vi "Impedance_Cryo_Configuration.vi"() -> ()   [LabVIEW 2018]
uses:
  <vilib>/Utility/file.llb/Write Delimited Spreadsheet (DBL).vi
  <instrlib>/Agilent 4194/Agilent 4194.lvlib
panel:
  in  "stop 2":bool
  in  "stop":bool
  in  "Start Impedance Collection":bool
  in  "Gain-Phase (0:Tch/Rch [dB] - Theta)":u32(ring) items=["Tch/Rch [dB] - Theta", "Tch/Rch - theta", "Tch/Rch [dB] - tau", "Tch-Rch [V]", "Tch-Rch [dBm]", "Tch-Rch [dBV]"]
  in  "Sweep Type (F:Linear)":bool
  in  "Stop/Span (10,00E-3)":dbl=15000000.0 format="%^.1e"
  in  "Start/Center (10,00E-3)":dbl=100.0 min=-40.0 max=40000000.0 format="%^.3e"
  in  "Display Mode (0:X - A&B)":u32(ring) items=["X - A&B", "A - B", "Table"]
  in  "Number Of Points (100)":i32=400 min=2 max=401
  in  "Averaging Number (8:256)":u32(ring) items=["1", "2", "4", "8", "16", "32", "64", "128", "256"]
  in  "Integration Time (0:Short)":u32(ring) items=["Short", "Medium", "Long"]
  in  "Impedance (0:| Z | - Theta )":u32(ring) items=["| Z | -Ttheta ", "R - X", "Ls-Rs", "Ls-Q", "Cs-Rs", "Cs-Q", "Cs-D", "|Y|-Theta", "G-B", "Lp-G", "Lp-Q", "Cp-G", "Cp-Q", "Cp-D", "|Z|-Ls", "|Z|-Cs", "|Z|-Lp", "|Z|-Cp", "Lp-Rp", "Cp-Rp"]
  in  "Measurement Type (0:Impedance)":u32(ring) items=["Impedance ", "Gain - Phase", "Impedance With Probe"]
  in  "File Base Name":string
  in  "error in (no error)":errorcluster
  in  "VISA resource name 2":refnum<visa-resource-name>="GPIB0::17::INSTR"
  out "A":T1(graph)
  out "B":T1(graph)
  out "error out":errorcluster
  in  "Force Quit":bool
  out "Status":string
  in  "Log Button In 4":bool
  in  "Log Button In 3":bool
  in  "Log Button In 2":bool
  in  "Log Button In 1":bool
  out "Input 4 Temperature Chart":dbl(graph)
  out "Input 3 Temperature Chart":dbl(graph)
  out "Input 1 Temperature Chart":dbl(graph)
  out "Input 2 Temperature Chart":dbl(graph)
  out "In 4 Value":dbl
  out "In 3 Value":dbl
  out "In 2 Value":dbl
  out "In 1 Value":dbl
  out "In 4 Channel Name":string
  out "In 3 Channel Name":string
  out "In 2 Channel Name":string
  out "In 1 Channel Name":string
  in  "VISA resource name":refnum<visa-resource-name>
  out "?":string
  out "?":string
  in  "Output 2":bool
  in  "Output 1":bool
  out "In 4 Channel Button Overlay":string
  out "In 3 Channel Button Overlay":string
  in  "Input 4 Button":bool
  in  "Input 3 Button":bool
  out "In 2 Channel Button Overlay":string
  out "In 1 Channel Button Overlay":string
  in  "Input 2 Button\nInput 2":bool
  in  "Input 1 Button":bool
  # "INPUT"
  # "OUTPUT"
  # "TEMPERATURE"
  # "K"
  # "K"
  # "K"
  # "K"
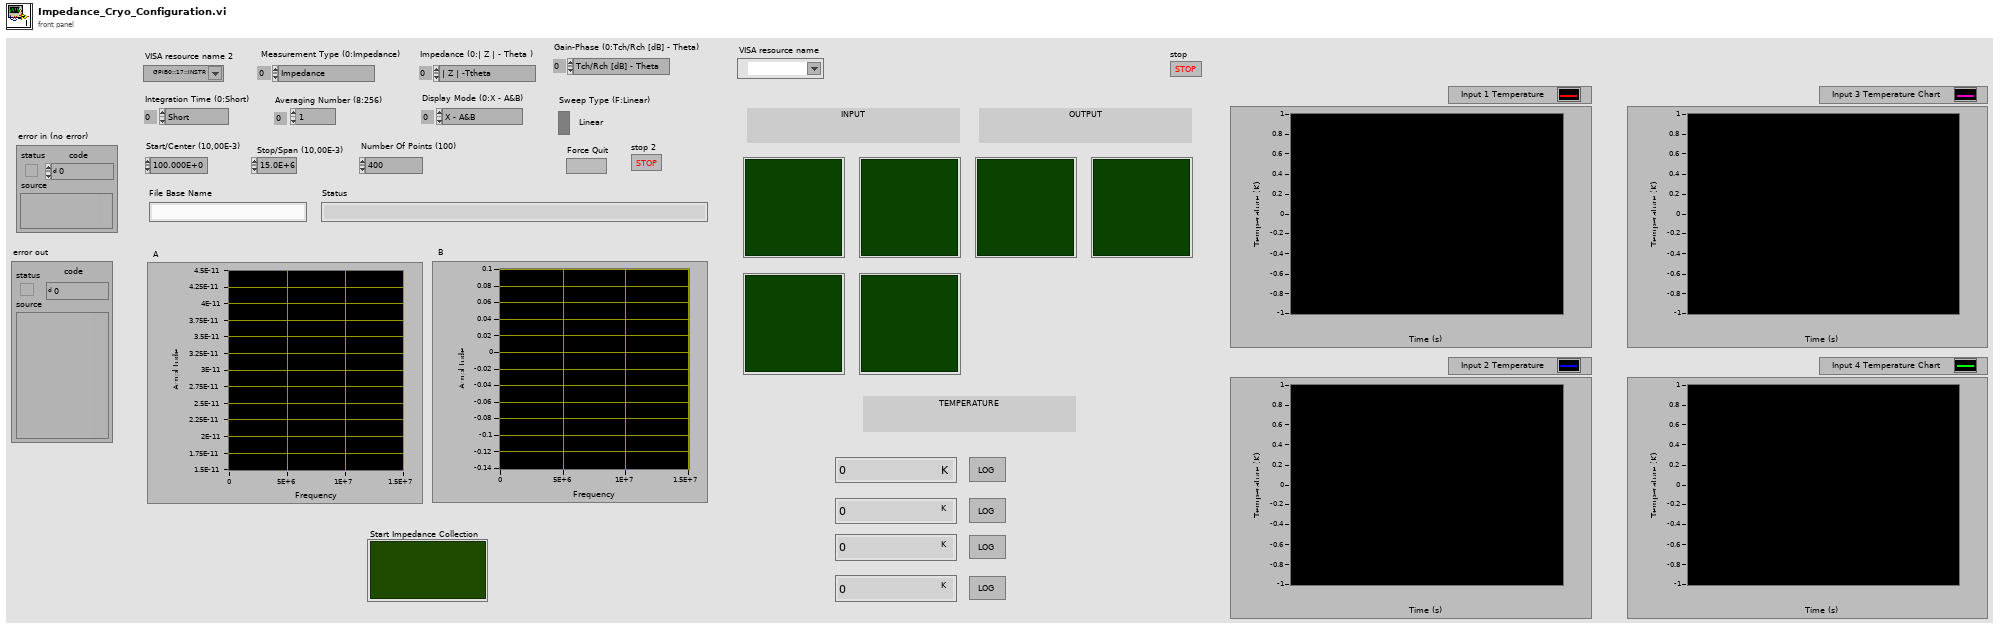
[diagram p1: front panel]
types:
  T1 = cluster{"Register Data":dbl[], "Offset/Calib Register Data":dbl[]}
  T2 = cluster{"[0]":dbl, "[1]":dbl, "[2]":dbl, "[3]":dbl, "[4]":dbl, "[5]":dbl, "[6]":dbl, "[7]":dbl, "[8]":dbl}
  T3 = cluster{"[0]":string, "[1]":string, "[2]":string, "[3]":string, "[4]":string, "[5]":string, "[6]":string, "[7]":string, "[8]":string}
  T4 = enum16{"open", "replace", "create", "open or create", "replace or create", "replace or create with confirmation"}
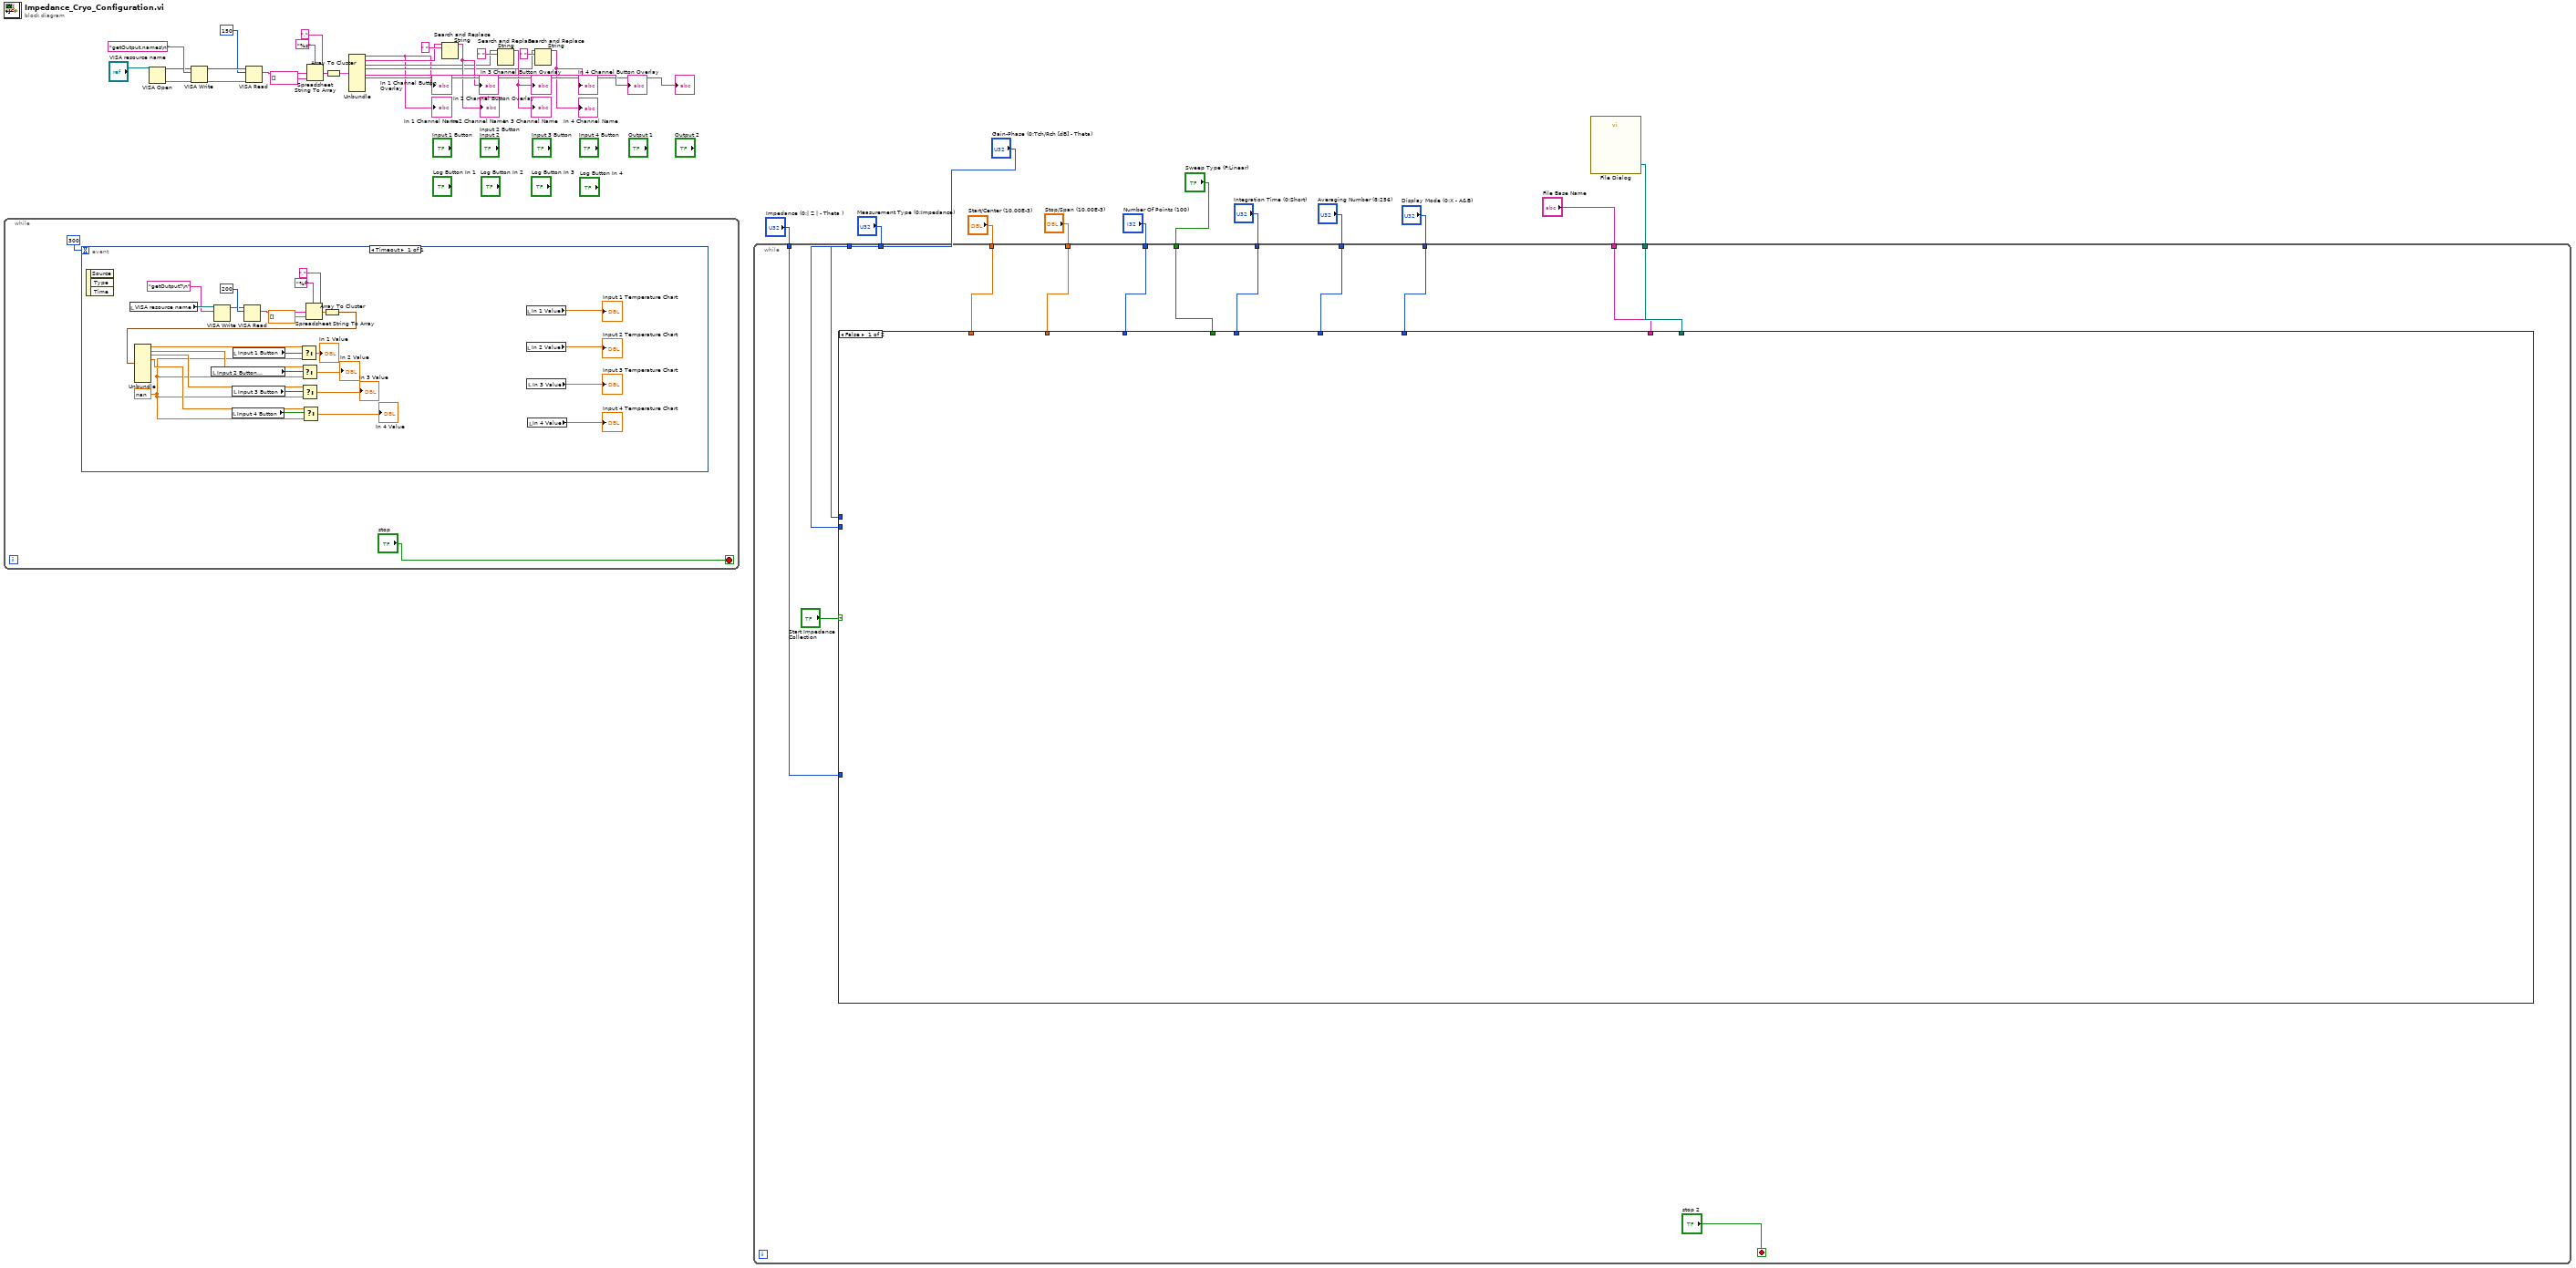
[diagram p0: block diagram]
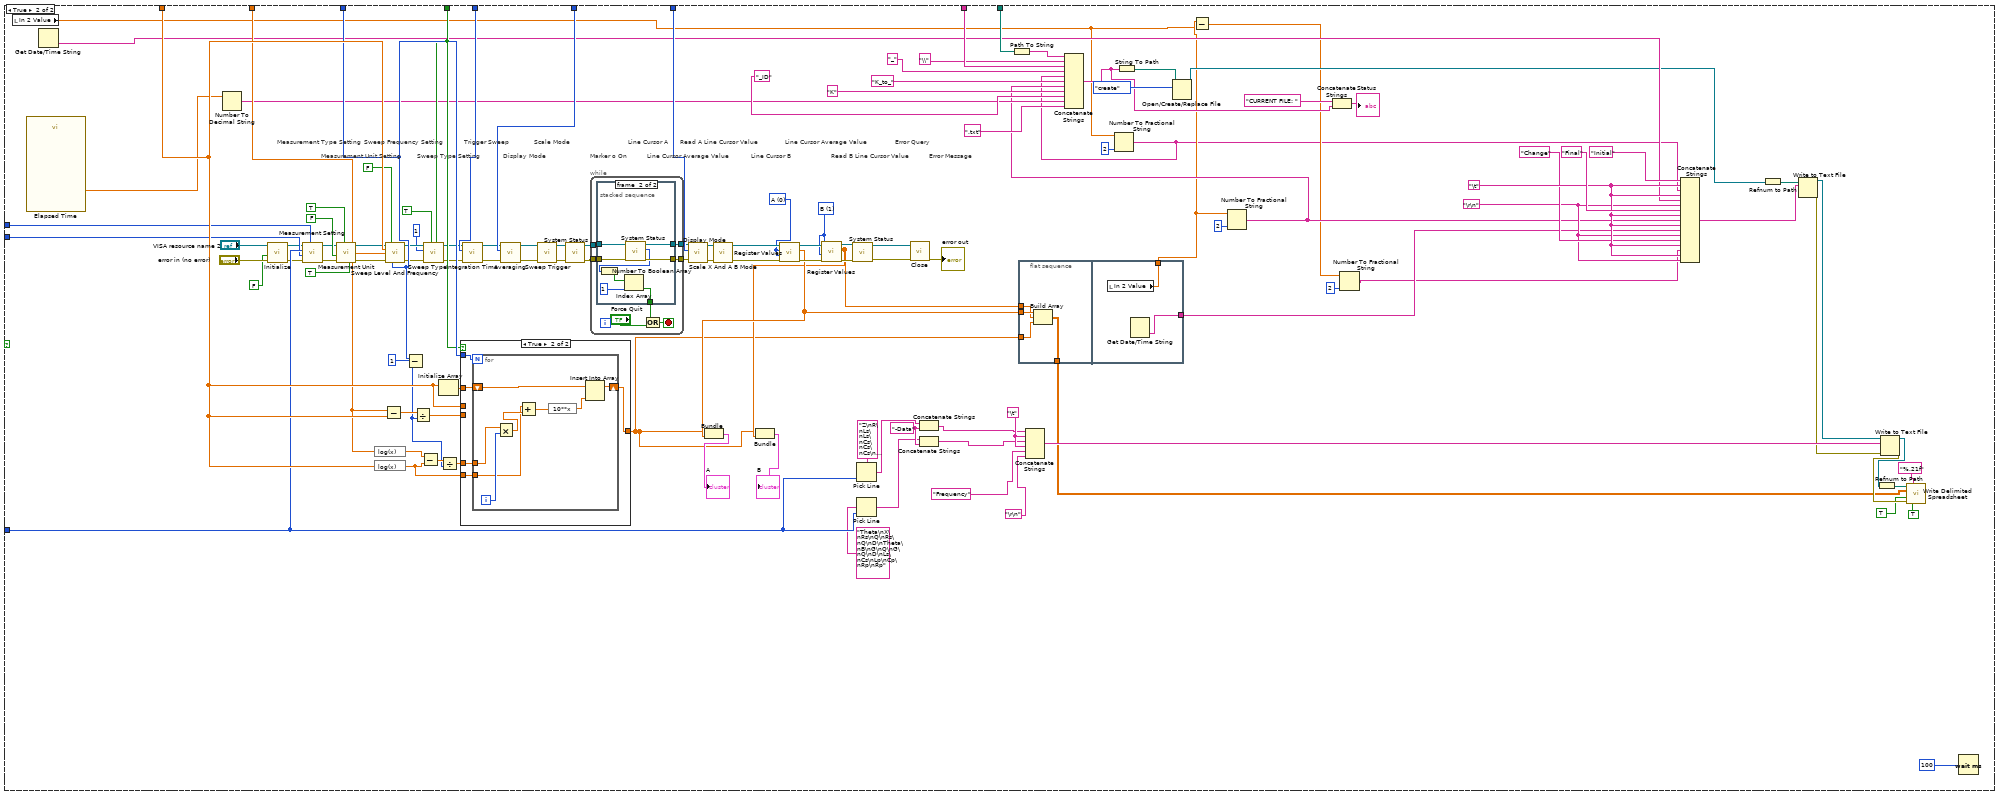
[diagram p2: hidden frame]
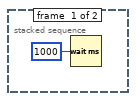
[diagram p3: hidden frame]
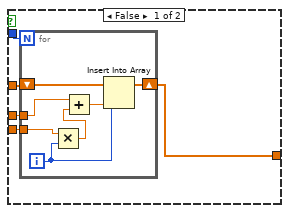
[diagram p4: hidden frame]
diagram:
  n1 = while {
    stop <- "stop" stop-if-true
    n2 = event shown="[0] Timeout" {
      selector: _ -> [_]
      dyn-events: _ -> [_]
      timeout: 300 -> [_]
      event Timeout {
        w49 = nan
        n3 = event-data() -> ()  [unwired: 1 in, 3 out]
        n4 = local read "VISA resource name"() -> (w66:refnum<visa-resource-name>)
        n5 = local read "Input 2 Button\nInput 2"() -> (w53:bool)
        n6 = VISA Write(VISA resource name=w66, write buffer="getOutput?\n") -> (VISA resource name out=w58:refnum<visa-resource-name>)  [unwired: 1 in, 2 out]
        n7 = local read "Input 4 Button"() -> (w48:bool)
        n8 = local read "Input 3 Button"() -> (w51:bool)
        n9 = local read "Input 1 Button"() -> (w55:bool)
        n10 = VISA Read(VISA resource name=w58, byte count=u32 200) -> (read buffer=w59:string)  [unwired: 1 in, 3 out]
        n11 = Spreadsheet String To Array(delimiter (Tab)=",", format string="%f", spreadsheet string=w59, array type (2D Dbl)=dbl[] []) -> (array=w61:dbl[])
        n12 = Array To Cluster(array=w61) -> (cluster=w57:T2)
        n13 = Unbundle(w57) -> ("[0]"=w56:dbl, "[1]"=w54:dbl, "[2]"=w52:dbl, "[3]"=w50:dbl)  [unwired: 5 out]
        n14 = Select(t=w56, s=w55, f=w49) -> (s? t:f=→"In 1 Value":dbl)
        n15 = Select(t=w54, s=w53, f=w49) -> (s? t:f=→"In 2 Value":dbl)
        n16 = Select(t=w52, s=w51, f=w49) -> (s? t:f=→"In 3 Value":dbl)
        n17 = Select(t=w50, s=w48, f=w49) -> (s? t:f=→"In 4 Value":dbl)
        n18 = local read "In 1 Value"() -> (→"Input 1 Temperature Chart":dbl)
        n19 = local read "In 2 Value"() -> (→"Input 2 Temperature Chart":dbl)
        n20 = local read "In 3 Value"() -> (→"Input 3 Temperature Chart":dbl)
        n21 = local read "In 4 Value"() -> (→"Input 4 Temperature Chart":dbl)
      }
    }
  }
  n22 = VISA Open(VISA resource name="VISA resource name") -> (VISA resource name=w13:refnum<visa-resource-name>, error out=w17:errorcluster)  [unwired: 4 in]
  n23 = VISA Write(VISA resource name=w13, write buffer="getOutput.names\n", error in (no error)=w17) -> (VISA resource name out=w20:refnum<visa-resource-name>, error out=w21:errorcluster)  [unwired: 1 out]
  n24 = VISA Read(VISA resource name=w20, byte count=u32 150, error in (no error)=w21) -> (read buffer=w15:string)  [unwired: 3 out]
  n25 = Spreadsheet String To Array(delimiter (Tab)=",", format string="%s", spreadsheet string=w15, array type (2D Dbl)=string[] []) -> (array=w31:string[])
  n26 = Array To Cluster(array=w31) -> (cluster=w34:T3)
  n27 = Unbundle(w34) -> ("[0]"=→"In 1 Channel Button Overlay" →"In 1 Channel Name":string, "[1]"=w29:string, "[2]"=w26:string, "[3]"=w23:string, "[4]"=→"?":string, "[5]"=→"?":string)  [unwired: 3 out]
  n28 = Search and Replace String(input string=w29, search string=" ") -> (result string=→"In 2 Channel Button Overlay" →"In 2 Channel Name":string)  [unwired: 6 in, 3 out]
  n29 = Search and Replace String(input string=w26, search string=" ") -> (result string=→"In 3 Channel Button Overlay" →"In 3 Channel Name":string)  [unwired: 6 in, 3 out]
  n30 = Search and Replace String(input string=w23, search string=" ") -> (result string=→"In 4 Channel Button Overlay" →"In 4 Channel Name":string)  [unwired: 6 in, 3 out]
  n31 = call "File Dialog"() -> ("selected path"=w5:path)  [unwired: 12 in, 3 out]
  n32 = while {
    tunnel: "Start/Center (10,00E-3)" -> [w80]
    tunnel: "Stop/Span (10,00E-3)" -> [w79]
    tunnel: "Number Of Points (100)" -> [w78]
    tunnel: "Sweep Type (F:Linear)" -> [w77]
    tunnel: "Integration Time (0:Short)" -> [w76]
    tunnel: "Averaging Number (8:256)" -> [w75]
    tunnel: "Display Mode (0:X - A&B)" -> [w74]
    tunnel: w5 -> [w73]
    tunnel: "File Base Name" -> [w72]
    tunnel: "Measurement Type (0:Impedance)" -> [w71]
    tunnel: "Impedance (0:| Z | - Theta )" -> [w70]
    tunnel: "Gain-Phase (0:Tch/Rch [dB] - Theta)" -> [w69]
    stop <- "stop 2" stop-if-true
    n33 = case shown="False" "Start Impedance Collection" {
      tunnel: w80 -> [_ w202]
      tunnel: w79 -> [_ w201]
      tunnel: w78 -> [_ w200]
      tunnel: w77 -> [_ w199]
      tunnel: w76 -> [_ w198]
      tunnel: w75 -> [_ w197]
      tunnel: w74 -> [_ w196]
      tunnel: w73 -> [_ w195]
      tunnel: w72 -> [_ w194]
      tunnel: w71 -> [_ w193]
      tunnel: w70 -> [_ w192]
      tunnel: w69 -> [_ w191]
      frame False {
      }
      frame True {
        w108 = "\r\n"
        w110 = "\t"
        w142 = "-Data" ("string")
        w145 = u32 0 items=["A", "B", "C", "D", "E", "F", "G", "H", "I", "J", "RA", "RB", "RC", "RD", "RE", "RF", "RG", "RH", "RI", "RJ", "RK", "RL"] ("Registers (0:A)")
        w149 = u32 1 items=["A", "B", "C", "D", "E", "F", "G", "H", "I", "J", "RA", "RB", "RC", "RD", "RE", "RF", "RG", "RH", "RI", "RJ", "RK", "RL"] ("Registers (0:A) 2")
        w148 = "\t"
        # "Error Message"
        # "Error Query"
        # "Line Cursor B"
        # "Line Cursor Average Value"
        # "Read B Line Cursor Value"
        # "Read A Line Cursor Value"
        # "Line Cursor Average Value"
        # "Line Cursor A"
        # "Marker o On"
        # "Scale Mode"
        # "Display Mode"
        # "Trigger Sweep"
        # "Sweep Type Setting"
        # "Sweep Frequency Setting"
        # "Measurement Unit Setting"
        # "Measurement Type Setting"
        n34 = local read "In 2 Value"() -> (w83:dbl)
        n35 = call "Elapsed Time"() -> ("Elapsed Time (s)"=w102:dbl)  [unwired: 12 in, 7 out]
        n36 = Get Date/Time String() -> (time string=w107:string)  [unwired: 3 in, 1 out]
        n37 = Number To Decimal String(number=w102) -> (decimal integer string=w98:string)  [unwired: 1 in]
        n38 = call <instrlib>:"Initialize.vi"("error in (no error)"="error in (no error)", "Reset Device (T:Reset Device)"=FALSE, "VISA resource name"="VISA resource name 2") -> ("error out"=w177:errorcluster, "VISA resource name out"=w176:refnum<visa-resource-name>)  [unwired: 7 in]
        n39 = call <instrlib>:"Measurement Setting.vi"("Measurement Type (0:Impedance)"=w193, "error in (no error)"=w177, "Gain-Phase (0:Tch/Rch [dB] - Theta)"=w191, "Impedance (0:| Z | - Theta )"=w192, "VISA resource name"=w176) -> ("error out"=w186:errorcluster, "VISA resource name out"=w187:refnum<visa-resource-name>)  [unwired: 5 in]
        n40 = call <instrlib>:"Measurement Unit.vi"("Test Input Impedance(T:50 ohm)"=TRUE ("Ref Attenuation (F:0 dB)"), "Power Splitter (F:Dual)"=TRUE ("Ref Attenuation (F:0 dB)"), "error in (no error)"=w186, "Ref Input Impedance (T:50 ohm)"=FALSE ("Ref Attenuation (F:0 dB)"), "VISA resource name"=w187) -> ("error out"=w184:errorcluster, "VISA resource name out"=w185:refnum<visa-resource-name>)  [unwired: 5 in]
        n41 = expression code="log(x)"(w201) -> (w155:dbl)
        n42 = expression code="log(x)"(w202) -> (w152:dbl)
        n43 = Subtract(x=w201, y=w202) -> (x-y=w165:dbl)
        n44 = call <instrlib>:"Sweep Level And Frequency.vi"("VISA resource name"=w185, "Step/Number Of Points (F:Points)"=FALSE ("Step/Number Of Points (F:Points))"), "Start/Center (10,00E-3)"=w202, "Stop/Span (10,00E-3)"=w201, "error in (no error)"=w184, "Number Of Points (100)"=w200) -> ("VISA resource name out"=w182:refnum<visa-resource-name>, "error out"=w181:errorcluster)  [unwired: 8 in]
        n45 = Subtract(x=w200, y=1) -> (x-y=w150:i32)
        n46 = Divide(x=w165, y=w150) -> (x/y=w164:dbl)
        n47 = Subtract(x=w155, y=w152) -> (x-y=w154:dbl)
        n48 = call <instrlib>:"Sweep Type.vi"("Sweep Type (F:Linear)"=w199, "Sweep Direction (F:Down)"=TRUE, "error in (no error)"=w181, "Sweep Mode (0:Repeat)"=u32 1, "VISA resource name"=w182) -> ("error out"=w172:errorcluster, "VISA resource name out"=w173:refnum<visa-resource-name>)  [unwired: 5 in]
        n49 = Initialize Array(w202) -> (w166:dbl[])  [unwired: 1 in]
        n50 = Divide(x=w154, y=w150) -> (x/y=w153:dbl)
        n51 = case shown="True" w199 {
          tunnel: w166 -> [w229 w240]
          tunnel: w200 -> [w228 w241]
          tunnel: w164 -> [w227 _]
          tunnel: w202 -> [w226 _]
          tunnel: [w225 w239] -> w92
          tunnel: w153 -> [_ w238]
          tunnel: w152 -> [_ w237]
          frame False {
            n52 = for {
              N: w228 -> [_]
              shift-right: [w235] -> w225
              shift-left: w229 -> [w236]
              tunnel: w226 -> [w232]
              tunnel: w227 -> [w230]
              i -> [w234]
              n53 = Multiply(x=w230, y=w234) -> (x*y=w231:dbl)
              n54 = Add(x=w232, y=w231) -> (x+y=w233:dbl)
              n55 = Insert Into Array(array=w236, index=w234, new element=w233) -> (w235:dbl[])
            }
          }
          frame True {
            n56 = for {
              N: w241 -> [_]
              shift-right: [w249] -> w239
              shift-left: w240 -> [w248]
              tunnel: w238 -> [w246]
              tunnel: w237 -> [w242]
              i -> [w245]
              n57 = Multiply(x=w246, y=w245) -> (x*y=w247:dbl)
              n58 = Add(x=w242, y=w247) -> (x+y=w244:dbl)
              n59 = expression code="10**x"(w244) -> (w243:dbl)
              n60 = Insert Into Array(array=w248, new element=w243) -> (w249:dbl[])  [unwired: 1 in]
            }
          }
        }
        n61 = call <instrlib>:"Integration Time.vi"("error in (no error)"=w172, "Integration Time (0:Short)"=w198, "VISA resource name"=w173) -> ("error out"=w170:errorcluster, "VISA resource name out"=w171:refnum<visa-resource-name>)  [unwired: 7 in]
        n62 = call <instrlib>:"Averaging.vi"("error in (no error)"=w170, "Averaging Number (8:256)"=w197, "VISA resource name"=w171) -> ("error out"=w168:errorcluster, "VISA resource name out"=w169:refnum<visa-resource-name>)  [unwired: 7 in]
        n63 = call <instrlib>:"Sweep Trigger.vi"("error in (no error)"=w168, "VISA resource name"=w169) -> ("error out"=w134:errorcluster, "VISA resource name out"=w135:refnum<visa-resource-name>)  [unwired: 8 in]
        n64 = call <instrlib>:"System Status.vi"("error in (no error)"=w134, "VISA resource name"=w135) -> ("error out"=w133:errorcluster, "VISA resource name out"=w132:refnum<visa-resource-name>)  [unwired: 6 in, 2 out]
        n65 = while {
          tunnel: w132 -> [w215]
          tunnel: w133 -> [w214]
          tunnel: [w213] -> w137
          tunnel: [w212] -> w136
          stop <- w211 stop-if-true
          n66 = stacked-sequence {
            tunnel: w215 -> [_ w224]
            tunnel: w214 -> [_ w223]
            tunnel: [_ w222] -> w213
            tunnel: [_ w221] -> w212
            tunnel: [_ w220] -> w209
            frame #0 {
              n67 = Wait (ms)(milliseconds to wait=u32 1000) -> ()  [unwired: 1 out]
            }
            frame #1 {
              n68 = call <instrlib>:"System Status.vi"("error in (no error)"=w223, "VISA resource name"=w224) -> ("error out"=w221:errorcluster, "ESR? (0)"=w219:i32, "VISA resource name out"=w222:refnum<visa-resource-name>)  [unwired: 6 in, 1 out]
              n69 = Number To Boolean Array(number=w219) -> (Boolean array=w218:bool[])
              n70 = Index Array(array=w218, index=1) -> (element=w220:bool)
            }
          }
          n71 = Or(x=w209, y="Force Quit") -> (x .or. y?=w211:bool)
        }
        n72 = call <instrlib>:"Display Mode.vi"("error in (no error)"=w136, "Display Mode (0:X - A&B)"=w196, "VISA resource name"=w137) -> ("error out"=w178:errorcluster, "VISA resource name out"=w179:refnum<visa-resource-name>)  [unwired: 7 in]
        n73 = call <instrlib>:"Scale X And A B Mode.vi"("VISA resource name"=w179, "error in (no error)"=w178) -> ("VISA resource name out"=w160:refnum<visa-resource-name>, "error out"=w159:errorcluster)  [unwired: 12 in]
        n74 = call <instrlib>:"Register Values.vi"("error in (no error)"=w159, "Calib/Offset Register (0:OFSTA)"=w145, "Registers (0:A)"=w145, "VISA resource name"=w160) -> ("error out"=w157:errorcluster, "Register Data"=w94:dbl[], "VISA resource name out"=w158:refnum<visa-resource-name>)  [unwired: 2 in, 3 out]
        n75 = Bundle(w92, "Register Data"=w94) -> (→"A":cluster{dbl[], "Register Data":dbl[]})  [unwired: 1 in]
        n76 = call <instrlib>:"Register Values.vi"("error in (no error)"=w157, "Calib/Offset Register (0:OFSTA)"=w149, "Registers (0:A)"=w149, "VISA resource name"=w158) -> ("error out"=w130:errorcluster, "Register Data"=w93:dbl[], "VISA resource name out"=w131:refnum<visa-resource-name>)  [unwired: 2 in, 3 out]
        n77 = Bundle(w92, "Register Data"=w93) -> (→"B":cluster{dbl[], "Register Data":dbl[]})  [unwired: 1 in]
        n78 = call <instrlib>:"System Status.vi"("error in (no error)"=w130, "VISA resource name"=w131) -> ("error out"=w128:errorcluster, "VISA resource name out"=w129:refnum<visa-resource-name>)  [unwired: 6 in, 2 out]
        n79 = Pick Line(multi-line string="Z\nR\nLs\nLs\nCs\nCs\nCs\nY\nG\nLp\nLp\nCp\nCp\nCp\nZ\nZ\nZ\nZ\nLp\nCp", line index=w192) -> (output string=w141:string)  [unwired: 1 in]
        n80 = Pick Line(multi-line string="Theta\nX\nRs\nQ\nRs\nQ\nD\nTheta\nB\nG\nQ\nG\nQ\nD\nLs\nCs\nLp\nCp\nRp\nRp", line index=w192) -> (output string=w140:string)  [unwired: 1 in]
        n81 = call <instrlib>:"Close.vi"("error in (no error)"=w128, "VISA resource name"=w129) -> ("error out"=→"error out":errorcluster)  [unwired: 9 in]
        n82 = Concatenate Strings(w141, w142) -> (w139:string)
        n83 = Concatenate Strings(w140, w142) -> (w138:string)
        n84 = Path To String(path=w195) -> (string=w127:string)
        n85 = flat-sequence {
          tunnel: w94 -> [w206]
          tunnel: w93 -> [w205]
          tunnel: w92 -> [w204]
          tunnel: [w203] -> w91
          tunnel: [w208] -> w88
          tunnel: [w207] -> w90
          frame #0 {
            n86 = Build Array(w206, w205, w204) -> (w203:dbl[][])
          }
          frame #1 {
            n87 = local read "In 2 Value"() -> (w208:dbl)
            n88 = Get Date/Time String() -> (time string=w207:string)  [unwired: 3 in, 1 out]
          }
        }
        n89 = Concatenate Strings(w139, w148, w138, w148, "Frequency" ("string"), "\r\n") -> (w117:string)
        n90 = Number To Fractional String(number=w83, precision (6)=i16 2) -> (F-format string=w82:string)  [unwired: 2 in]
        n91 = Subtract(x=w88, y=w83) -> (x-y=w85:dbl)
        n92 = Number To Fractional String(number=w88, precision (6)=i16 2) -> (F-format string=w89:string)  [unwired: 2 in]
        n93 = Concatenate Strings(w127, "\\", w194, "_", w82, "K_to_" ("string"), w89, "K" ("string"), "_ID", w98, ".txt" ("string")) -> (w95:string)
        n94 = String To Path(string=w95) -> (path=w125:path)
        n95 = Open/Create/Replace File(file path (use dialog)=w125, operation (0:open)=T4."create") -> (refnum out=w106:refnum<file>)  [unwired: 4 in, 2 out]
        n96 = Concatenate Strings("CURRENT FILE: " ("string"), w95) -> (→"Status":string)
        n97 = Number To Fractional String(number=w85, precision (6)=i16 2) -> (F-format string=w86:string)  [unwired: 2 in]
        n98 = Concatenate Strings("Initial" ("string"), w110, w82, w110, w107, w108, "Final" ("string"), w110, w89, w110, w90, w108, "Change" ("string"), w110, w86, w110, w108) -> (w104:string)
        n99 = Refnum to Path(1:w106) -> (0:w105:path)
        n100 = Write to Text File(file (use dialog)=w105, text=w104) -> (refnum out=w96:refnum<file>, error out=w103:errorcluster)  [unwired: 2 in, 1 out]
        n101 = Write to Text File(file (use dialog)=w96, text=w117, error in=w103) -> (refnum out=w120:refnum<file>, error out=w119:errorcluster)  [unwired: 1 in, 1 out]
        n102 = Refnum to Path(1:w120) -> (0:w121:path)
        n103 = call-poly <vilib>:"Write Delimited Spreadsheet.vi"("file path (dialog if empty)"=w121, "format (%.3f)"="%.21f", "2D data"=w91, "append to file? (new file:F)"=TRUE ("append to file? (F)"), "error in (no error)"=w119, "transpose? (no:F)"=TRUE ("transpose? (F)")) -> ()  [unwired: 8 in, 2 out]
        n104 = Wait (ms)(milliseconds to wait=u32 100) -> ()  [unwired: 1 out]
      }
    }
  }
